vi "Get status Response.vi"(8 "error in (no error)":errorcluster, 11 "Cypress in":refnum<class "Cypress.lvclass">) -> (0 "error out":errorcluster, 2 "Response":string, 3 "Cypress out":refnum<class "Cypress.lvclass">)   [LabVIEW 2020, in "Cypress.lvclass"]
uses:
  Cypress.lvclass
  Abstracts/Serial Device/Serial Device.lvclass
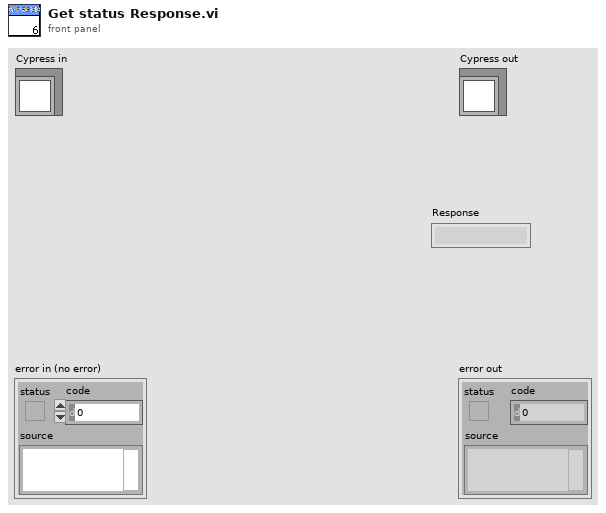
[diagram p1: front panel]
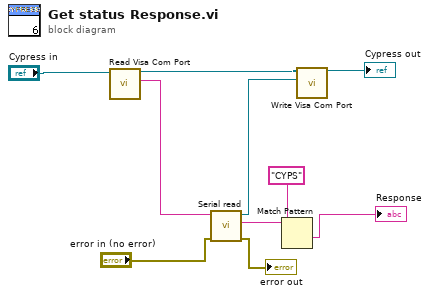
[diagram p0: block diagram]
diagram:
  n1 = call-dynamic "Read Visa Com Port.vi"("Serial Device in"="Cypress in") -> ("Visa Com Port"=w7:string, "Serial Device out"=w8:refnum<class "Cypress.lvclass">)  [unwired: 8 in, 1 out]
  n2 = call "Serial read.vi"("error in (no error)"="error in (no error)", "VISA resource name in"=w7) -> ("error out"=→"error out":errorcluster, "Respuesta"=w3:string, "VISA resource name out"=w4:refnum<visa-resource-name>)  [unwired: 7 in]
  n3 = Match Pattern(string=w3, regular expression="CYPS") -> (after substring=→"Response":string)  [unwired: 1 in, 3 out]
  n4 = call-dynamic "Write Visa Com Port.vi"("Visa Com Port"=w4, "Serial Device in"=w8) -> ("Serial Device out"=→"Cypress out":refnum<class "Cypress.lvclass">)  [unwired: 8 in, 1 out]
